vi "Read actCtl.vi"(8 "error in (no error)":errorcluster, 11 "AlicatCommBank in":refnum<class "AlicatCommBank.lvclass">=refnum) -> (0 "error out":errorcluster, 2 "actCtl":string, 3 "AlicatCommBank out":refnum<class "AlicatCommBank.lvclass">)   [LabVIEW 2014, in "Alicat.lvlib" / "AlicatCommBank.lvclass"]
uses:
  AlicatCommBank.lvclass
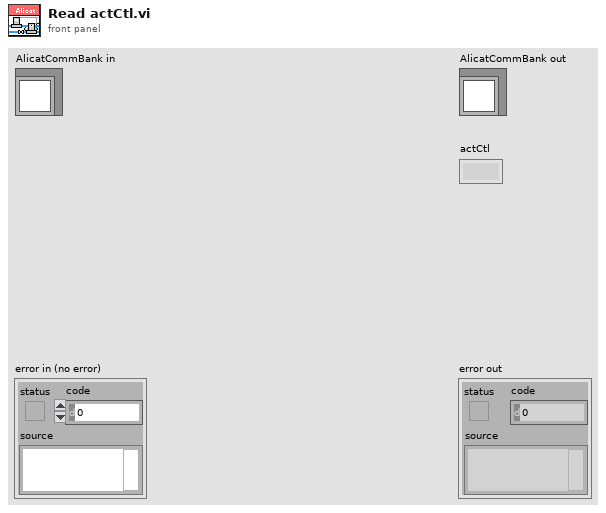
[diagram p1: front panel]
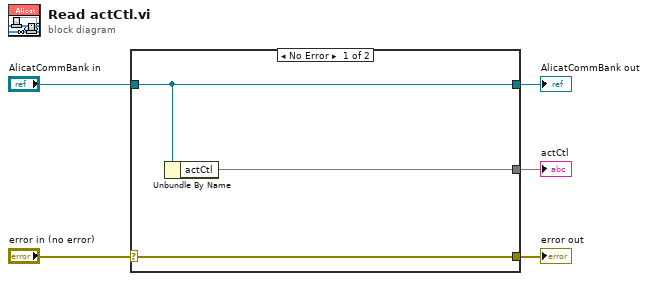
[diagram p0: block diagram]
diagram:
  n1 = case shown="No Error" "error in (no error)" {
    selector: "error in (no error)" -> [w8 w9]
    tunnel: [w8 w9] -> w4
    tunnel: [w7 w10] -> w2
    tunnel: "AlicatCommBank in" -> [w7 w10]
    tunnel: [w6 _] -> w1
    frame No Error {
      n2 = Unbundle By Name(w7) -> ("actCtl"=w6)
    }
    frame Error {
    }
  }
  "error out" <- w4
  "AlicatCommBank out" <- w2
  "actCtl" <- w1
